vi "Load Store Macro.vi"(7 "File Name":string, 8 "error in (no error)":errorcluster, 9 "Macro Name":string, 10 "Operation Type (0: Load)":i32(ring) items=["Load", "Store"], 11 "VISA resource name":refnum<visa-resource-name>) -> (0 "error out":errorcluster, 3 "VISA resource name out":refnum<visa-resource-name>)   [LabVIEW 2012, in "Keysight B2980 Series.lvlib"]
doc: "Loads or saves the macro from or to the specified file in the current directory."
uses:
  Keysight B2980 Series.lvlib
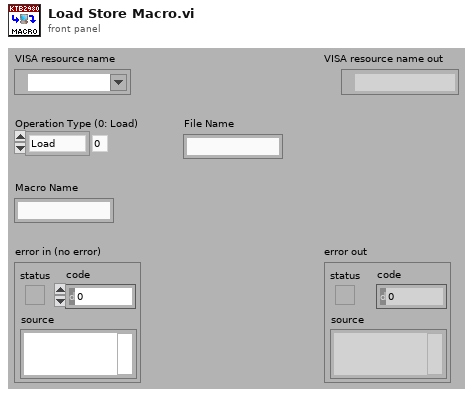
[diagram p1: front panel]
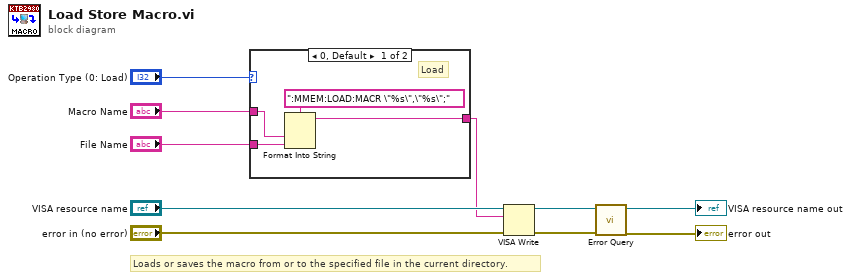
[diagram p0: block diagram]
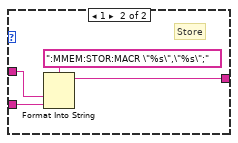
[diagram p2: hidden frame]
diagram:
  # "Loads or saves the macro from or to the specified file in the current directory."
  n1 = case shown="0, Default" "Operation Type (0: Load)" {
    tunnel: "Macro Name" -> [w13 w16]
    tunnel: "File Name" -> [w12 w17]
    tunnel: [w11 w15] -> w1
    frame 0, Default {
      # "Load"
      n2 = Format Into String(format string=":MMEM:LOAD:MACR \"%s\",\"%s\";", w13, w12) -> (resulting string=w11:string)  [unwired: 2 in, 1 out]
    }
    frame 1 {
      # "Store"
      n3 = Format Into String(format string=":MMEM:STOR:MACR \"%s\",\"%s\";", w16, w17) -> (resulting string=w15:string)  [unwired: 2 in, 1 out]
    }
  }
  n4 = VISA Write(VISA resource name="VISA resource name", write buffer=w1, error in (no error)="error in (no error)") -> (VISA resource name out=w8:refnum<visa-resource-name>, error out=w7:errorcluster)  [unwired: 1 out]
  n5 = call "Error Query.vi"("error in (no error)"=w7, "VISA resource name"=w8) -> ("error out"=→"error out":errorcluster, "VISA resource name out"=→"VISA resource name out":refnum<visa-resource-name>)  [unwired: 8 out]
